vi "process_image.vi"(0 "Image Processing Data In":T2, 2 "Raw Image Data In":T4, 7 "Threshold range":cluster{"Lower value":sgl, "Upper value":sgl}={"Lower value"=6.0, "Upper value"=1024.0}, 11 "error in (no error)":errorcluster) -> (4 "Image Processing Data Out":T2, 8 "Output data":T1, 13 "Number of Particles":u16, 15 "error out":errorcluster)   [LabVIEW 2023]
uses:
  <vilib>/vision/Image Controls.llb/IMAQ Image.ctl
  <vilib>/vision/NI_Vision_Development_Module.lvlib
panel:
  out "Image Data Out":T4
  out "Particle Measurements (Pixels)":dbl[][](array[numeric])
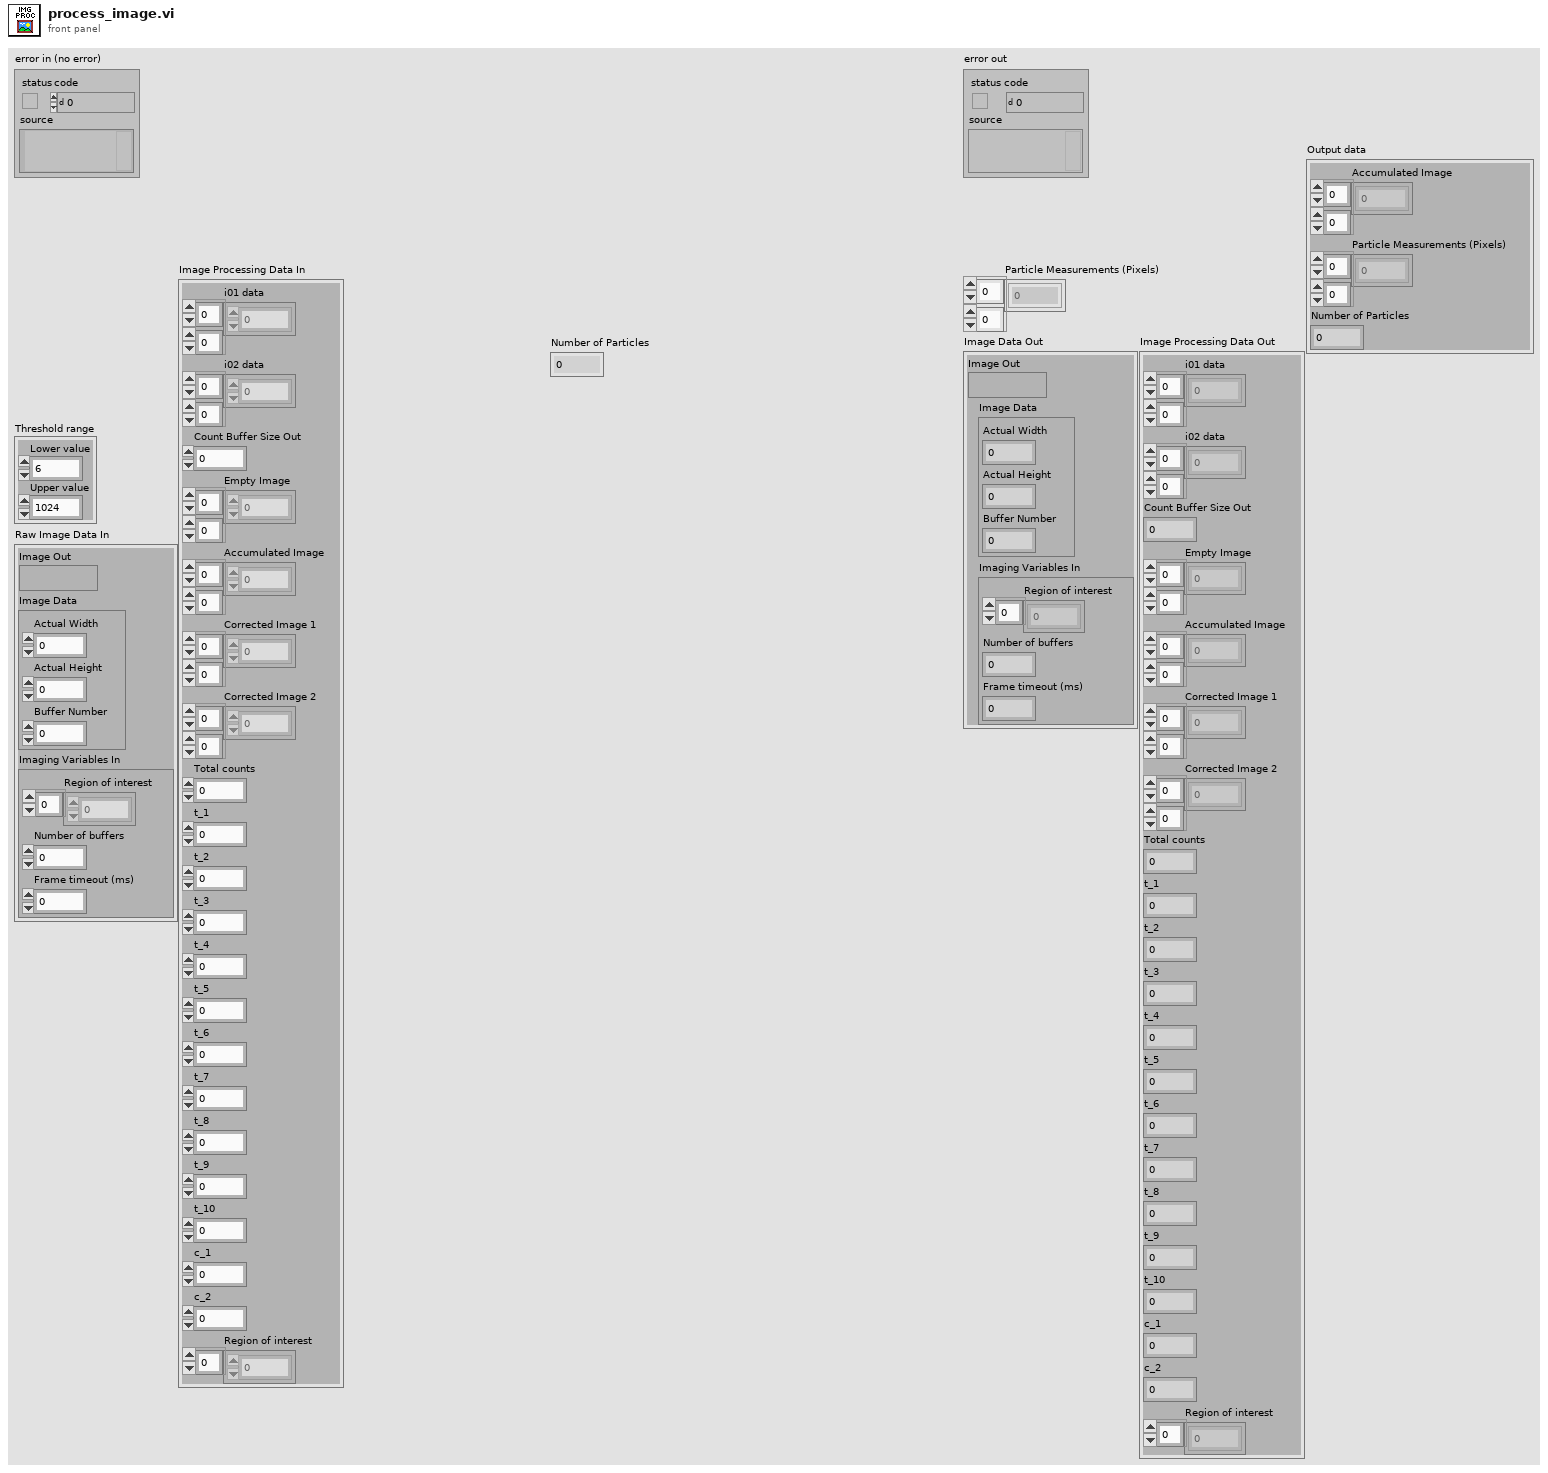
[diagram p1: front panel]
types:
  T1 = cluster{"Accumulated Image":i16[][], "Particle Measurements (Pixels)":dbl[][], "Number of Particles":u16}
  T2 = cluster{"i01 data":sgl[][], "i02 data":sgl[][], "Count Buffer Size Out":i32, "Empty Image":i16[][], "Accumulated Image":i16[][], "Corrected Image 1":i16[][], "Corrected Image 2":i16[][], "Total counts":i32, "t_1":i32, "t_2":i32, "t_3":i32, "t_4":i32, "t_5":i32, "t_6":i32, "t_7":i32, "t_8":i32, "t_9":i32, "t_10":i32, "c_1":i32, "c_2":i32, "Region of interest":i32[]}
  T3 = typedef "IMAQ Image.ctl" = refnum<image>
  T4 = cluster{"Image Out":T3, "Image Data":cluster{"Actual Width":u32, "Actual Height":u32, "Buffer Number":i32}, "Imaging Variables In":cluster{"Region of interest":i32[], "Number of buffers":u32, "Frame timeout (ms)":u32}}
  T5 = typedef "Particle Parameters" = i32
  T6 = enum32{"AutoM", "Close", "Dilate", "Erode", "Gradient", "Gradient in", "Gradient out", "HitMiss", "Open", "PClose", "POpen", "Thick", "Thin"}
  T7 = cluster{"Accumulated Image":i16[][], "Particle Measurements (Pixels)":dbl[][], "Number of Particles":i32}
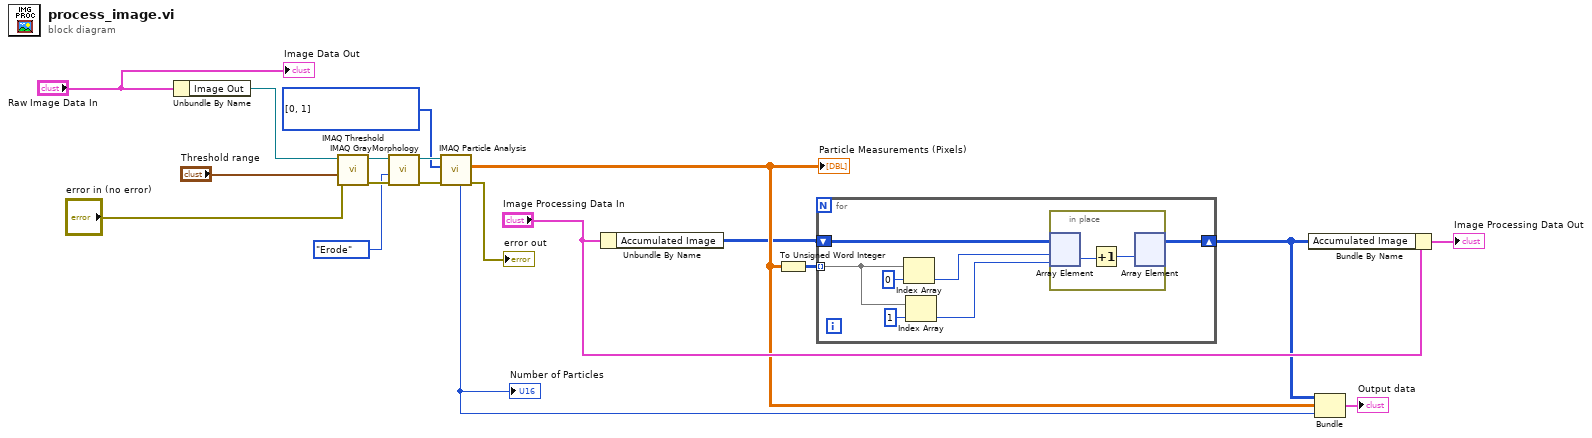
[diagram p0: block diagram]
diagram:
  w7 = T5[] [0, 1] items=["Center of Mass X", "Center of Mass Y", "First Pixel X", "First Pixel Y", "Bounding Rect Left", "Bounding Rect Top", "Bounding Rect Right", "Bounding Rect Bottom", "Max Feret Diameter Start X", "Max Feret Diameter Start Y", "Max Feret Diameter End X", "Max Feret Diameter End Y", "Max Horiz. Segment Length Left", "Max Horiz. Segment Length Right", "Max Horiz. Segment Length Row", "-", "Bounding Rect Width", "Bounding Rect Height", "Bounding Rect Diagonal", "Perimeter", "Convex Hull Perimeter", "Holes' Perimeter", "Max Feret Diameter", "Equivalent Ellipse Major Axis", "Equivalent Ellipse Minor Axis", "Equivalent Ellipse Minor Axis (Feret)", "Equivalent Rect Long Side", "Equivalent Rect Short Side", "Equivalent Rect Diagonal", "Equivalent Rect Short Side (Feret)", "Average Horiz. Segment Length", "Average Vert. Segment Length", "Hydraulic Radius", "Waddel Disk Diameter", "-", "Area", "Holes' Area", "Particle & Holes' Area", "Convex Hull Area", "Image Area", "-", "Number of Holes", "Number of Horiz. Segments", "Number of Vert. Segments", "-", "Orientation", "Max Feret Diameter Orientation", "-", "% Area/Image Area", "% Area/(Particle & Holes' Area)", "Ratio of Equivalent Ellipse Axes", "Ratio of Equivalent Rect Sides", "-", "Elongation Factor", "Compactness Factor", "Heywood Circularity Factor", "Type Factor", "-", "Sum X", "Sum Y", "Sum XX", "Sum XY", "Sum YY", "Sum XXX", "Sum XXY", "Sum XYY", "Sum YYY", "-", "Moment of Inertia XX", "Moment of Inertia XY", "Moment of Inertia YY", "Moment of Inertia XXX", "Moment of Inertia XXY", "Moment of Inertia XYY", "Moment of Inertia YYY", "Norm. Moment of Inertia XX", "Norm. Moment of Inertia XY", "Norm. Moment of Inertia YY", "Norm. Moment of Inertia XXX", "Norm. Moment of Inertia XXY", "Norm. Moment of Inertia XYY", "Norm. Moment of Inertia YYY", "Hu Moment 1", "Hu Moment 2", "Hu Moment 3", "Hu Moment 4", "Hu Moment 5", "Hu Moment 6", "Hu Moment 7"] ("Pixel Measurements")
  n1 = Unbundle By Name("Raw Image Data In") -> ("Image Out"=w9:T3)
  n2 = call "IMAQ Threshold"("error in (no error)"="error in (no error)", "Range"="Threshold range", "Image Src"=w9) -> ("error out"=w12:errorcluster, "Image Dst Out"=w14:T3)  [unwired: 7 in]
  n3 = call "IMAQ GrayMorphology"("error in (no error)"=w12, "Operation"=T6."Erode", "Image Src"=w14) -> ("error out"=w11:errorcluster, "Image Dst Out"=w13:T3)  [unwired: 7 in]
  n4 = call "IMAQ Particle Analysis"("error in (no error)"=w11, "Pixel Measurements"=w7, "Image"=w13) -> ("error out"=→"error out":errorcluster, "Particle Measurements (Pixels)"=w5:dbl[][], "Number of Particles"=w6:i32)  [unwired: 3 in, 3 out]
  "Number of Particles" <- w6
  "Particle Measurements (Pixels)" <- w5
  n5 = Unbundle By Name("Image Processing Data In") -> ("Accumulated Image"=w3:i16[][])
  n6 = To Unsigned Word Integer(number=w5) -> (unsigned 16bit integer=w19:u16[][])
  n7 = for {
    tunnel: w19 -> [w25] mode=indexing
    shift-right: [w22] -> w1
    shift-left: w3 -> [w23]
    n8 = Index Array(array=w25, index=0) -> (element=w21:u16)
    n9 = Index Array(array=w25, index=1) -> (element=w20:u16)
    n10 = in-place {
      n11 = in-place-array #1(w23, w21, w20) -> (w28:i16)
      n12 = Increment(x=w28) -> (x+1=w27:i16)
      n13 = in-place-array #1(w27) -> (w22:i16[][])  [unwired: 2 out]
    }
  }
  n14 = Bundle By Name(cluster="Image Processing Data In", "Accumulated Image"=w1) -> (→"Image Processing Data Out":T2)
  n15 = Bundle("Accumulated Image"=w1, "Particle Measurements (Pixels)"=w5, "Number of Particles"=w6) -> (→"Output data":T7)  [unwired: 1 in]
  "Image Data Out" <- "Raw Image Data In"
